vi "Player Info.vi"(11 "Class":refnum<class "Spawn.lvclass">) -> (0 "Defeat Speech":string, 1 "Victory Speech":string, 2 "Name":string, 3 "Class":refnum<class "Spawn.lvclass">)   [LabVIEW 2020, in "Spawn.lvclass"]
uses:
  Spawn.lvclass
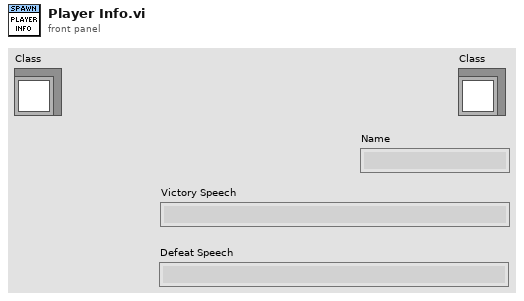
[diagram p1: front panel]
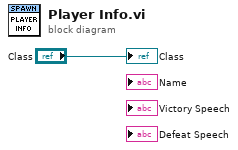
[diagram p0: block diagram]
diagram:
  "Class" <- "Class"
